vi "Set 2D Ramp Rates_entwurf.vi"(0 "Y-Axis Communications Config":T1={"GPIB address"=22, "GPIB bus"=0, "connection ID"=refnum, "IP"="192.168.2.200", "Active Comm Interface"=0, "Serial Port"="", "Programmer Type"=0} {"Programmer Type" items=["Model 430", "Model 420"]; "Active Comm Interface" items=["TCP/IP (Model 430 Only)", "RS232", "IEEE488"]}, 1 "Y-Axis Field (kG)":dbl format="%.3f", 3 "Next Y-Axis Field (kG)":dbl format="%.3f", 4 "Z-Axis Communications Config":T1={"GPIB address"=22, "GPIB bus"=0, "connection ID"=refnum, "IP"="192.168.2.200", "Active Comm Interface"=0, "Serial Port"="", "Programmer Type"=0} {"Programmer Type" items=["Model 430", "Model 420"]; "Active Comm Interface" items=["TCP/IP (Model 430 Only)", "RS232", "IEEE488"]}, 5 "Z-Axis Field (kG)":dbl format="%.3f", 6 "User defined Ramp Rate (T/min)":bool, 7 "Next Z-Axis Field (kG)":dbl format="%.3f", 8 "Max Ramp Rate - Y Axis (A/s)":dbl format="%.3f", 9 "Max Ramp Rate - Z Axis (A/s)":dbl format="%.3f", 10 "User defined Ramp Rate - Z Axis (kG/s)":dbl format="%.3f", 11 "error in":T2, 12 "User defined Ramp Rate Y-Axis (kG/s)":dbl format="%.3f") -> (15 "Y-Axis Ramp Rate (T/min)":dbl format="%.3f", 17 "Z-Axis Ramp Rate (T/min)":dbl format="%.3f", 18 "error out":T2)   [LabVIEW 2009]
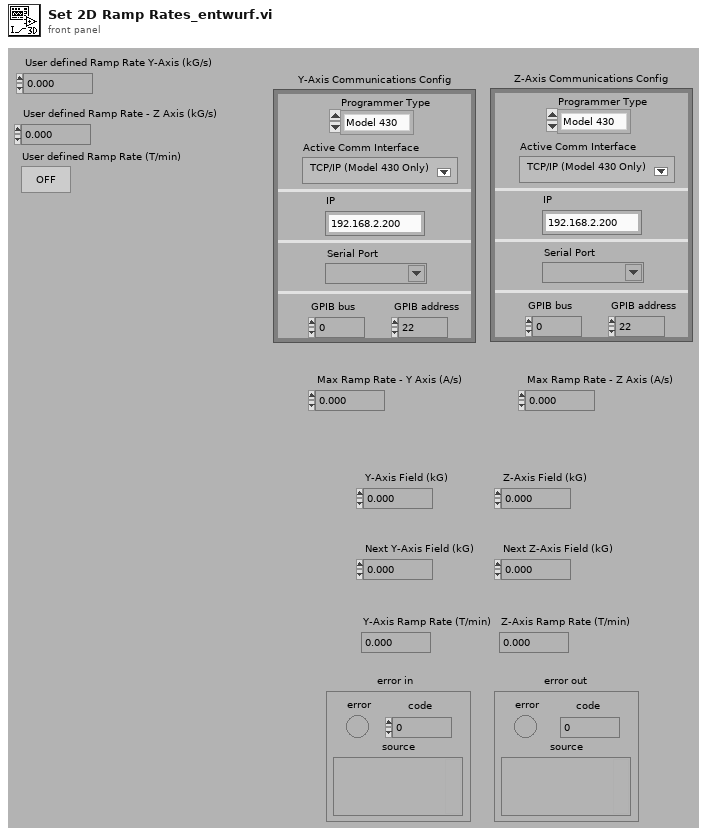
[diagram p1: front panel]
types:
  T1 = cluster{"GPIB address":i16, "GPIB bus":i16, "connection ID":refnum<k5>, "IP":string, "Active Comm Interface":u16, "Serial Port":refnum<visa-resource-name>, "Programmer Type":u16}
  T2 = cluster{"error":bool, "code":i32, "source":string}
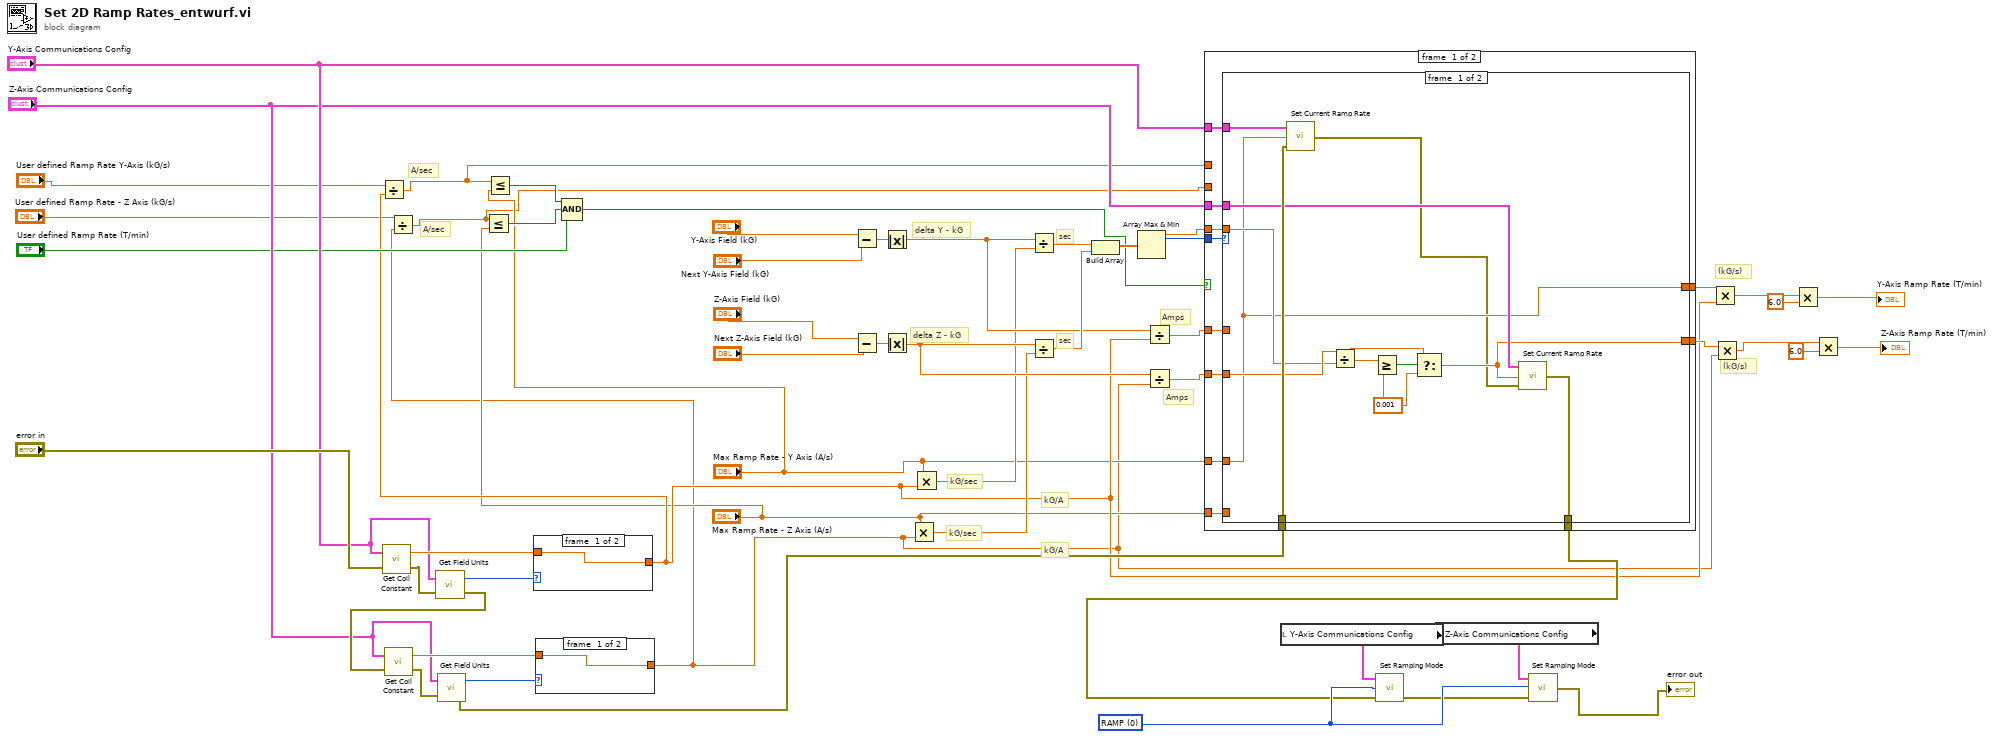
[diagram p0: block diagram]
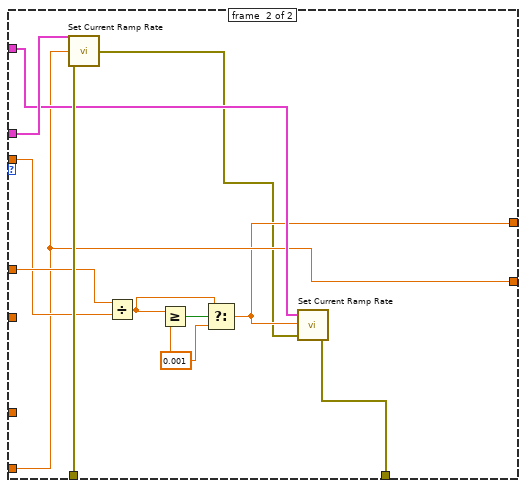
[diagram p2: hidden frame]
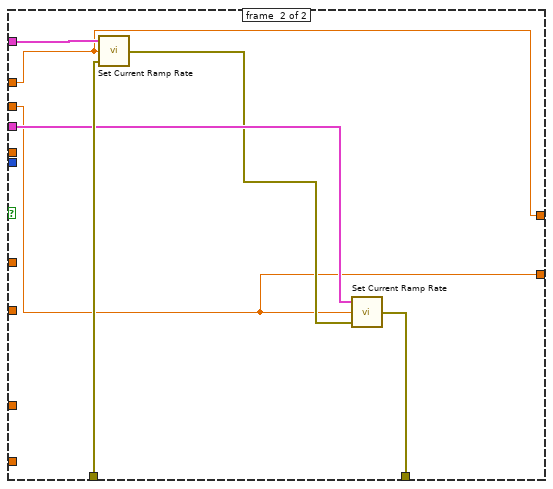
[diagram p3: hidden frame]
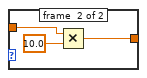
[diagram p4: hidden frame]
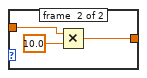
[diagram p5: hidden frame]
diagram:
  w37 = u16 0 items=["RAMP", "PAUSE", "MANUAL UP", "MANUAL DOWN", "ZERO"] ("Ramping Mode")
  # "(kG/s)"
  # "(kG/s)"
  # "A/sec"
  # "A/sec"
  # "Amps"
  # "Amps"
  # "kG/A"
  # "kG/A"
  # "kG/sec"
  # "kG/sec"
  # "delta Z - kG"
  # "delta Y - kG"
  # "sec"
  # "sec"
  n1 = call <userlib>:"Get Coil Constant.vi"("error in"="error in", "Communications Config"="Y-Axis Communications Config") -> ("error out"=w30:T2, "Coil Constant"=w31:dbl)
  n2 = call <userlib>:"Get Field Units.vi"("error in"=w30, "Communications Config"="Y-Axis Communications Config") -> ("error out"=w26:T2, "Field Units"=w32:enum16{"kg", "t"})
  n3 = call <userlib>:"Get Coil Constant.vi"("error in"=w26, "Communications Config"="Z-Axis Communications Config") -> ("error out"=w27:T2, "Coil Constant"=w28:dbl)
  n4 = call <userlib>:"Get Field Units.vi"("error in"=w27, "Communications Config"="Z-Axis Communications Config") -> ("error out"=w25:T2, "Field Units"=w29:enum16{"kg", "t"})
  n5 = case shown="\"t\"" w32 {
    tunnel: w31 -> [w55 w57]
    tunnel: [w55 w56] -> w12
    frame #0 {
    }
    frame #1 {
      n6 = Multiply(x=w57, y=10.0) -> (x*y=w56:dbl)
    }
  }
  n7 = Divide(x="User defined Ramp Rate Y-Axis (kG/s)", y=w12) -> (x/y=w13:dbl)
  n8 = Less Or Equal?(x=w13, y="Max Ramp Rate - Y Axis (A/s)") -> (x <= y?=w18:bool)
  n9 = case shown="\"t\"" w29 {
    tunnel: w28 -> [w59 w61]
    tunnel: [w59 w60] -> w8
    frame #0 {
    }
    frame #1 {
      n10 = Multiply(x=w61, y=10.0) -> (x*y=w60:dbl)
    }
  }
  n11 = Divide(x="User defined Ramp Rate - Z Axis (kG/s)", y=w8) -> (x/y=w7:dbl)
  n12 = Less Or Equal?(x=w7, y="Max Ramp Rate - Z Axis (A/s)") -> (x <= y?=w17:bool)
  n13 = Compound Arithmetic op=AND(w18, w17, "User defined Ramp Rate (T/min)") -> (w15:bool)
  n14 = Subtract(x="Y-Axis Field (kG)", y="Next Y-Axis Field (kG)") -> (x-y=w47:dbl)
  n15 = Subtract(x="Z-Axis Field (kG)", y="Next Z-Axis Field (kG)") -> (x-y=w46:dbl)
  n16 = Absolute Value(x=w47) -> (abs(x)=w44:dbl)
  n17 = Absolute Value(x=w46) -> (abs(x)=w43:dbl)
  n18 = Multiply(x="Max Ramp Rate - Z Axis (A/s)", y=w8) -> (x*y=w20:dbl)
  n19 = Multiply(x="Max Ramp Rate - Y Axis (A/s)", y=w12) -> (x*y=w19:dbl)
  n20 = Divide(x=w44, y=w19) -> (x/y=w54:dbl)
  n21 = Divide(x=w43, y=w20) -> (x/y=w53:dbl)
  n22 = Build Array(w54, w53) -> (w45:dbl[])
  n23 = Array Max & Min(array=w45) -> (max value=w42:dbl, max index (indices)=w48:i32)  [unwired: 2 out]
  n24 = Divide(x=w44, y=w12) -> (x/y=w41:dbl)
  n25 = Divide(x=w43, y=w8) -> (x/y=w40:dbl)
  n26 = case shown="True" w15 {
    tunnel: w48 -> [w74 _]
    tunnel: w42 -> [w73 _]
    tunnel: w41 -> [w72 _]
    tunnel: w40 -> [w71 _]
    tunnel: [w70 w100] -> w39
    tunnel: [w69 w99] -> w38
    tunnel: w25 -> [w68 w105]
    tunnel: "Max Ramp Rate - Y Axis (A/s)" -> [w67 _]
    tunnel: "Max Ramp Rate - Z Axis (A/s)" -> [w66 _]
    tunnel: [w65 w104] -> w23
    tunnel: "Y-Axis Communications Config" -> [w64 w103]
    tunnel: "Z-Axis Communications Config" -> [w63 w102]
    tunnel: w13 -> [_ w100]
    tunnel: w7 -> [_ w99]
    frame #0 {
      n27 = case shown="0, Default" w74 {
        tunnel: w68 -> [w85 w97]
        tunnel: w73 -> [w83 w95]
        tunnel: w72 -> [_ w96]
        tunnel: w64 -> [w86 w94]
        tunnel: w71 -> [w84 _]
        tunnel: w63 -> [w82 w98]
        tunnel: [w81 w93] -> w65
        tunnel: [w80 w88] -> w70
        tunnel: [w76 w92] -> w69
        tunnel: w67 -> [w80 _]
        tunnel: w66 -> [_ w92]
        frame #0 {
          w79 = 0.001 ("f")
          n28 = call <userlib>:"Set Current Ramp Rate.vi"("Communications Config"=w86, "Ramp Rate (A/sec)"=w80, "error in"=w85) -> ("error out"=w75:T2)  [unwired: 2 in]
          n29 = Divide(x=w84, y=w83) -> (x/y=w77:dbl)
          n30 = Greater Or Equal?(x=w77, y=w79) -> (x >= y?=w78:bool)
          n31 = Select(t=w77, s=w78, f=w79) -> (s? t:f=w76:dbl)
          n32 = call <userlib>:"Set Current Ramp Rate.vi"("Communications Config"=w82, "Ramp Rate (A/sec)"=w76, "error in"=w75) -> ("error out"=w81:T2)  [unwired: 2 in]
        }
        frame #1 {
          w91 = 0.001 ("f")
          n33 = call <userlib>:"Set Current Ramp Rate.vi"("Communications Config"=w98, "Ramp Rate (A/sec)"=w92, "error in"=w97) -> ("error out"=w87:T2)  [unwired: 2 in]
          n34 = Divide(x=w96, y=w95) -> (x/y=w89:dbl)
          n35 = Greater Or Equal?(x=w89, y=w91) -> (x >= y?=w90:bool)
          n36 = Select(t=w89, s=w90, f=w91) -> (s? t:f=w88:dbl)
          n37 = call <userlib>:"Set Current Ramp Rate.vi"("Communications Config"=w94, "Ramp Rate (A/sec)"=w88, "error in"=w87) -> ("error out"=w93:T2)  [unwired: 2 in]
        }
      }
    }
    frame #1 {
      n38 = call <userlib>:"Set Current Ramp Rate.vi"("Communications Config"=w103, "Ramp Rate (A/sec)"=w100, "error in"=w105) -> ("error out"=w101:T2)  [unwired: 2 in]
      n39 = call <userlib>:"Set Current Ramp Rate.vi"("Communications Config"=w102, "Ramp Rate (A/sec)"=w99, "error in"=w101) -> ("error out"=w104:T2)  [unwired: 2 in]
    }
  }
  n40 = local read "Y-Axis Communications Config"() -> (w35:T1)
  n41 = call <userlib>:"Set Ramping Mode.vi"("error in"=w23, "Ramping Mode"=w37, "Communications Config"=w35) -> ("error out"=w36:T2)
  n42 = local read "Z-Axis Communications Config"() -> (w34:T1)
  n43 = call <userlib>:"Set Ramping Mode.vi"("error in"=w36, "Ramping Mode"=w37, "Communications Config"=w34) -> ("error out"=→"error out":T2)
  n44 = Multiply(x=w39, y=w12) -> (x*y=w3:dbl)
  n45 = Multiply(x=w38, y=w8) -> (x*y=w6:dbl)
  n46 = Multiply(x=w3, y=6.0) -> (x*y=→"Y-Axis Ramp Rate (T/min)":dbl)
  n47 = Multiply(x=w6, y=6.0) -> (x*y=→"Z-Axis Ramp Rate (T/min)":dbl)
